vi "Byte Buffer.Write (SGL).vi"(8 "error in (no error)":errorcluster, 9 "value":sgl, 10 "buffer offset":u64, 11 "Byte Buffer in":refnum<class "Byte Buffer.lvclass">) -> (0 "error out":errorcluster, 2 "new buffer offset":u64, 3 "Byte Buffer out":refnum<class "Byte Buffer.lvclass">)   [LabVIEW 2016, in "VeriStand Data.lvlib" / "Byte Buffer.lvclass"]
doc: "Writes <B>value</B> to the provided <B>Byte Buffer</B> at location <B>buffer offset</B> in the format of the data type specified."
uses:
  Byte Buffer.lvclass
  Byte Buffer.lvclass/Byte Buffer.ctl
  Byte Buffer.Subset.Set.vi
  Byte Buffer.Get Buffer Pointer.vi
  Byte Buffer.Get Buffer Size.vi
  Memory Management/Memory Management.MoveByteBlock.Read (String).vi
  Memory Management/Memory Management.Handle Return.vi
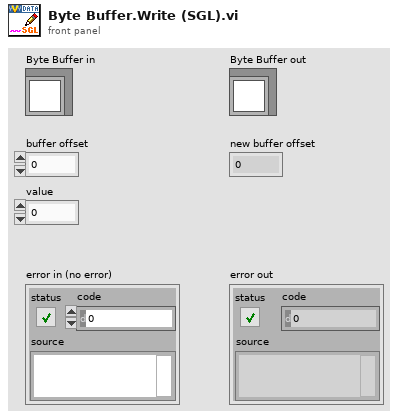
[diagram p1: front panel]
types:
  T1 = enum16{"big-endian, network order", "native, host order", "little-endian"}
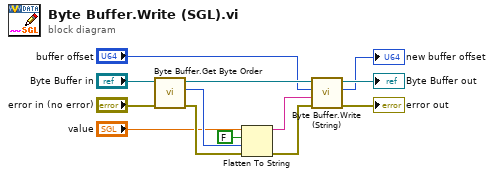
[diagram p0: block diagram]
diagram:
  n1 = call "Byte Buffer.Get Byte Order.vi"("error in (no error)"="error in (no error)", "Byte Buffer in"="Byte Buffer in") -> ("error out"=w9:errorcluster, "byte order"=w8:T1, "Byte Buffer out"=w10:refnum<class "Byte Buffer.lvclass">)  [unwired: 7 in]
  n2 = Flatten To String(anything="value", prepend array or string size? (T)=FALSE, byte order (0:big-endian, network order)=w8, error in (no error)=w9) -> (data string=w11:string, error out=w12:errorcluster)  [unwired: 1 out]
  n3 = call "Byte Buffer.Write (String).vi"("error in (no error)"=w12, "string"=w11, "buffer offset"="buffer offset", "Byte Buffer in"=w10) -> ("error out"=→"error out":errorcluster, "new buffer offset"=→"new buffer offset":u64, "Byte Buffer out"=→"Byte Buffer out":refnum<class "Byte Buffer.lvclass">)  [unwired: 5 in]
